vi "Sentuator_OS5000US.vi"(0 "VISA resource name":refnum<visa-resource-name>, 2 "Text to prepend to sentence":string="\n", 3 "error in (no error)":errorcluster) -> (4 "Angles":dbl[][](graph), 5 "VISA resource name out":refnum<visa-resource-name>, 6 "Remaining Sentence":string, 7 "error out":errorcluster)   [LabVIEW 2012]
uses:
  <instrlib>/Ocean Server OS4000/Ocean Server OS4000.lvlib
panel:
  in  "Send Output Rate":bool
  in  "Send Filter Value":bool
  in  "Send Mount Orientation":bool
  in  "Send Declination":bool
  in  "Output Rate":dbl
  in  "Average Samples":i32
  in  "Analog to Digital Conversion":i32
  in  "Mount Orientation (Default-Flat)":i32(ring)=1
  in  "Degauss Every":i32
  in  "Send Degauss":bool
  in  "Declination Angle":i32
  in  "Check Error":bool
  out "Error?":bool
  out "rollAngle":dbl
  out "pitchAngle":dbl
  out "compassHeading":dbl
  out "Mx":dbl
  out "My":dbl
  out "Mz":dbl
  out "Temperature":dbl
  out "Gyro X":dbl
  out "Gyro Y":dbl
  out "yAccel":dbl
  out "xAccel":dbl
  out "zAccel":dbl
  out "Magnetic Field":dbl[][](graph)
  out "Accel":dbl[][](graph)
  out "Temp":dbl[][](graph)
  out "Gyro":dbl[][](graph)
  out "Acceleration":dbl caption="Acceleration Magnitude"
  out "Magnetic Vector Field":dbl
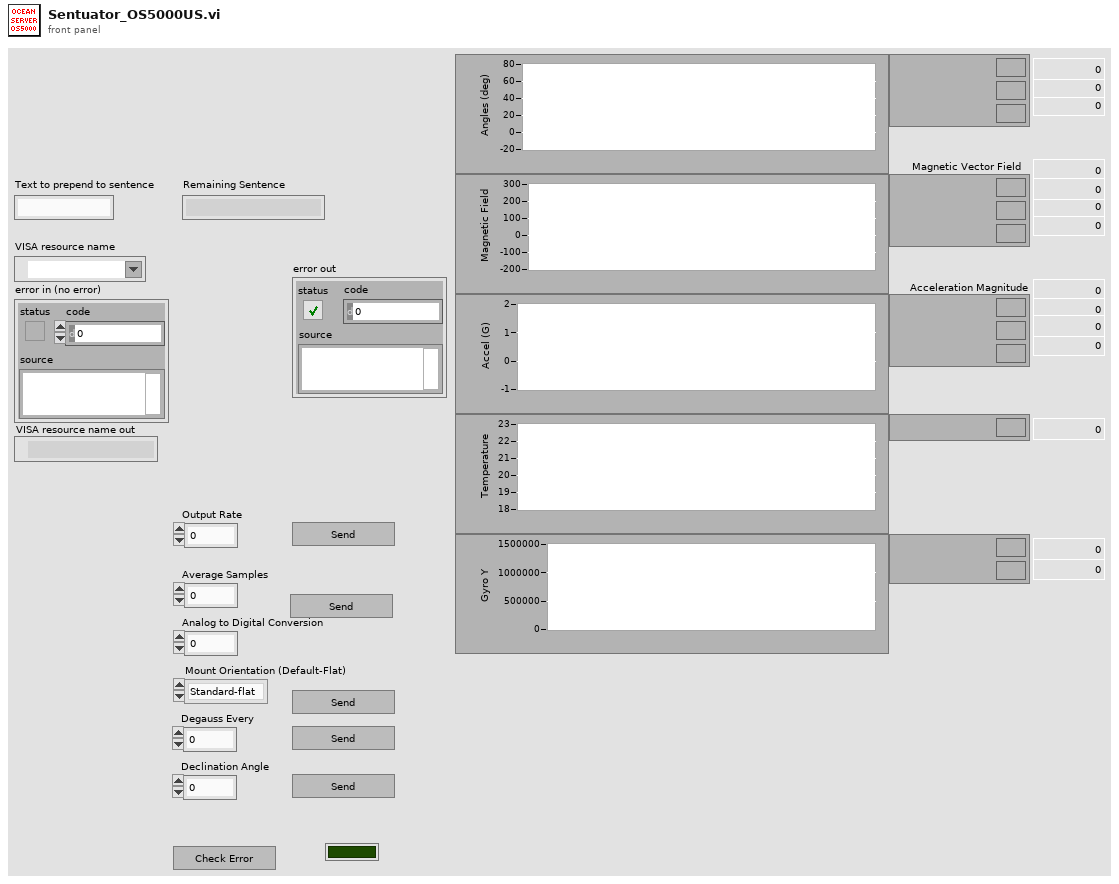
[diagram p1: front panel]
types:
  T1 = cluster{"Compass Heading":dbl, "pitch Angle":dbl, "roll Angle":dbl, "Temperature":dbl, "Depth":dbl, "Magnetic Field":dbl, "Magnetic Field X":dbl, "Magnetic Field Y":dbl, "Magnetic Field Z":dbl, "Acceleration":dbl, "Acceleration X":dbl, "Acceleration Y":dbl, "Gyro":dbl, "Gyro X":dbl, "Acceleration Z":dbl, "Gyro Y":dbl}
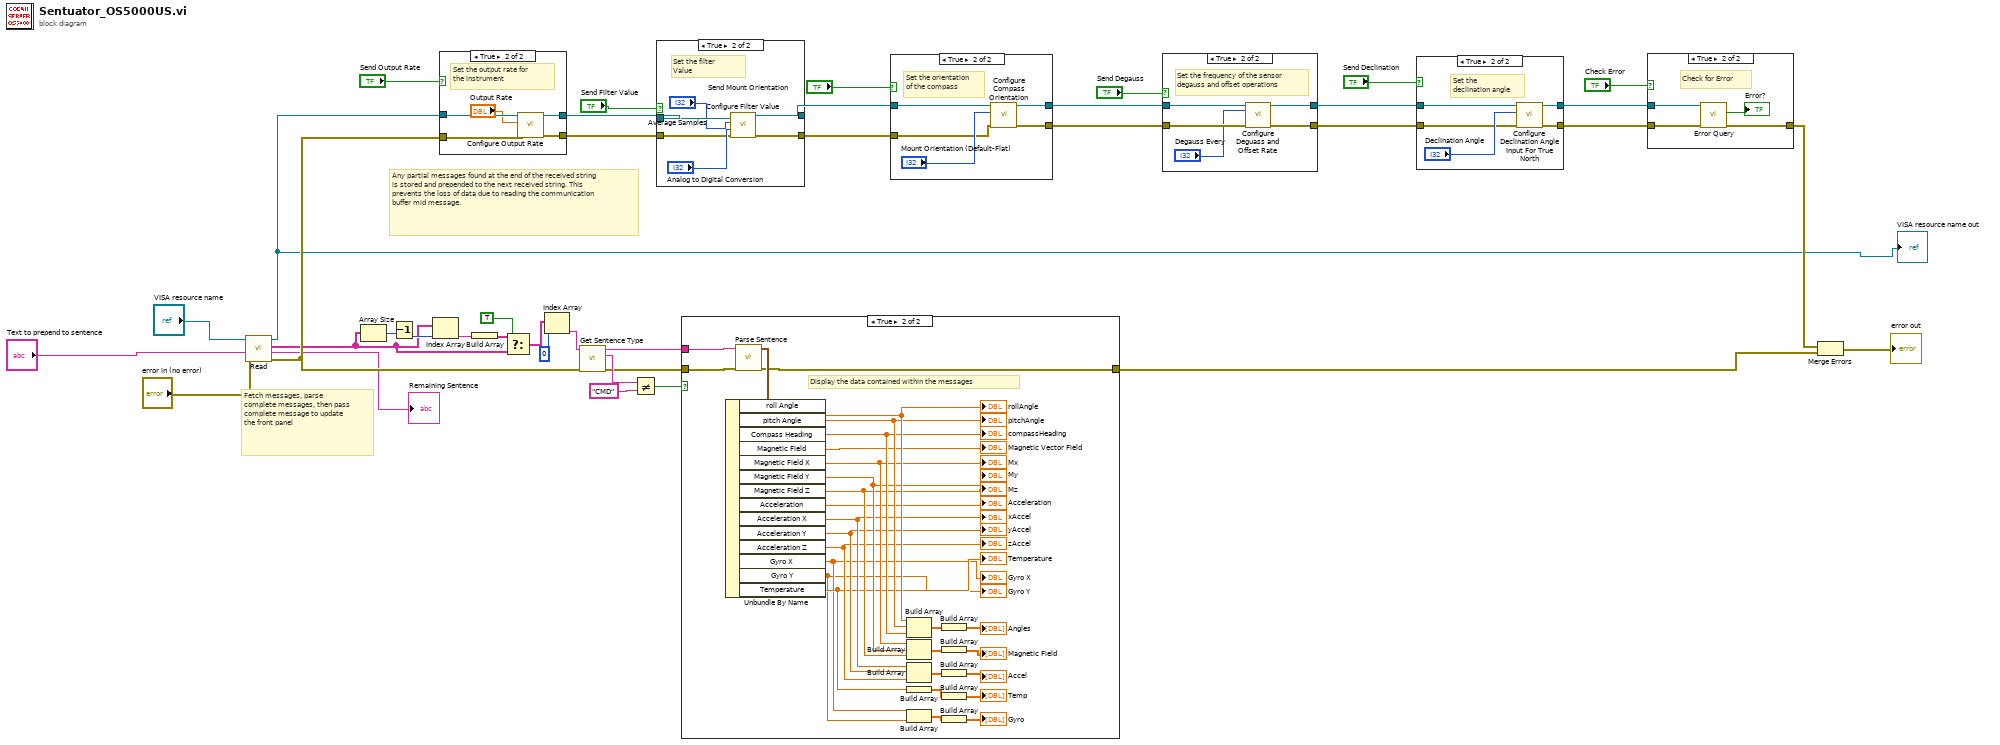
[diagram p0: block diagram]
diagram:
  # "Any partial messages found at the end of the received string is stored and prepended to the next received string. This prevents the loss of data due to reading the communication buffer mid message."
  # "Fetch messages, parse complete messages, then pass  complete message to update the front panel"
  n1 = call <instrlib>:"Read.vi"("error in (no error)"="error in (no error)", "Text to prepend to sentence"="Text to prepend to sentence", "VISA resource name"="VISA resource name") -> ("error out"=w27:errorcluster, "Remaining Sentence"=→"Remaining Sentence":string, "Ocean Server Sentences"=w16:string[], "VISA resource name out"=w7:refnum<visa-resource-name>)  [unwired: 5 in]
  "VISA resource name out" <- w7
  n2 = Array Size(array=w16) -> (size(s)=w20:i32)
  n3 = Decrement(x=w20) -> (x-1=w19:i32)
  n4 = Index Array(array=w16, index=w19) -> (element=w18:string)
  n5 = case shown="True" "Send Output Rate" {
    tunnel: w7 -> [w41 w46]
    tunnel: [w41 w44] -> w38
    tunnel: [w40 w43] -> w30
    tunnel: w27 -> [w40 w42]
    frame False {
    }
    frame True {
      # "Set the output rate for the instrument"
      n6 = call <instrlib>:"Configure Output Rate.vi"("Error in (no error)"=w42, "Output Rate ( 4 )"="Output Rate", "VISA resource name"=w46) -> ("Error out"=w43:errorcluster, "VISA resource out"=w44:refnum<visa-resource-name>)  [unwired: 7 in]
    }
  }
  n7 = Build Array(w18) -> (w17:string[])
  n8 = Select(t=w17, s=TRUE, f=w16) -> (s? t:f=w6:string[])
  n9 = Index Array(array=w6, index=0) -> (element=w4:string)
  n10 = call <instrlib>:"Get Sentence Type.vi"("error in (no error)"=w27, "Sentence In"=w4) -> ("error out"=w10:errorcluster, "Sentence Type"=w14:string, "Sentence Out"=w11:string)  [unwired: 7 in]
  n11 = Not Equal?(x=w14, y="CMD") -> (x != y?=w12:bool)
  n12 = case shown="True" "Send Filter Value" {
    tunnel: w38 -> [w48 w54]
    tunnel: [w48 w51] -> w36
    tunnel: w30 -> [w47 w50]
    tunnel: [w47 w49] -> w29
    frame False {
    }
    frame True {
      # "Set the filter Value"
      n13 = call <instrlib>:"Configure Filter Value.vi"("error in (no error)"=w50, "Filter Value for Analog to Digital Conversion ( 3 )"="Analog to Digital Conversion", "Averaging Value ( 4 )"="Average Samples", "VISA resource name"=w54) -> ("error out"=w49:errorcluster, "VISA resource out"=w51:refnum<visa-resource-name>)  [unwired: 6 in]
    }
  }
  n14 = case shown="True" w12 {
    tunnel: w11 -> [_ w59]
    tunnel: w10 -> [w55 w56]
    tunnel: [w55 w57] -> w21
    frame False {
      # "Front Panel isn't updated if the message received is not of the N1 type"
    }
    frame True {
      # "Display the data contained within the messages"
      n15 = call <instrlib>:"Parse Sentence.vi"("error in (no error)"=w56, "Ocean Server Sentence"=w59) -> ("error out"=w57:errorcluster, "Values"=w58:T1)  [unwired: 8 in]
      n16 = Unbundle By Name(w58) -> ("roll Angle"=w83:dbl, "pitch Angle"=w82:dbl, "Compass Heading"=w81:dbl, "Magnetic Field"=→"Magnetic Vector Field":dbl, "Magnetic Field X"=w80:dbl, "Magnetic Field Y"=w79:dbl, "Magnetic Field Z"=w78:dbl, "Acceleration"=→"Acceleration":dbl, "Acceleration X"=w77:dbl, "Acceleration Y"=w76:dbl, "Acceleration Z"=w75:dbl, "Gyro X"=w72:dbl, "Gyro Y"=w71:dbl, "Temperature"=w74:dbl)
      "rollAngle" <- w83
      "pitchAngle" <- w82
      "compassHeading" <- w81
      "Mx" <- w80
      "My" <- w79
      "Mz" <- w78
      "Temperature" <- w74
      "Gyro X" <- w72
      "Gyro Y" <- w71
      "yAccel" <- w76
      "xAccel" <- w77
      "zAccel" <- w75
      n17 = Build Array(w83, w82, w81) -> (w67:dbl[])
      n18 = Build Array(w80, w79, w78) -> (w68:dbl[])
      n19 = Build Array(w77, w76, w75) -> (w69:dbl[])
      n20 = Build Array(w74) -> (w73:dbl[])
      n21 = Build Array(w72, w71) -> (w70:dbl[])
      n22 = Build Array(w67) -> (→"Angles":dbl[][])
      n23 = Build Array(w68) -> (→"Magnetic Field":dbl[][])
      n24 = Build Array(w69) -> (→"Accel":dbl[][])
      n25 = Build Array(w73) -> (→"Temp":dbl[][])
      n26 = Build Array(w70) -> (→"Gyro":dbl[][])
    }
  }
  n27 = case shown="True" "Send Mount Orientation" {
    tunnel: w36 -> [w85 w89]
    tunnel: [w85 w88] -> w34
    tunnel: w29 -> [w84 w87]
    tunnel: [w84 w86] -> w28
    frame False {
    }
    frame True {
      # "Set the orientation of the compass"
      n28 = call <instrlib>:"Configure Compass Orientation.vi"("error in (no error)"=w87, "Mount Orientation ( Flat )"="Mount Orientation (Default-Flat)", "VISA resource name"=w89) -> ("error out"=w86:errorcluster, "VISA resource out"=w88:refnum<visa-resource-name>)  [unwired: 7 in]
    }
  }
  n29 = case shown="True" "Send Degauss" {
    tunnel: w34 -> [w92 w97]
    tunnel: [w92 w96] -> w33
    tunnel: [w91 w95] -> w32
    tunnel: w28 -> [w91 w94]
    frame False {
    }
    frame True {
      # "Set the frequency of the sensor degauss and offset operations"
      n30 = call <instrlib>:"Configure Deguass and Offset Rate.vi"("error in (no error)"=w94, "Deguass and Offset Rate ( 1 )"="Degauss Every", "VISA resource name"=w97) -> ("error out"=w95:errorcluster, "VISA resource out"=w96:refnum<visa-resource-name>)  [unwired: 7 in]
    }
  }
  n31 = case shown="True" "Send Declination" {
    tunnel: w33 -> [w99 w103]
    tunnel: w32 -> [w98 w102]
    tunnel: [w99 w101] -> w25
    tunnel: [w98 w100] -> w24
    frame False {
    }
    frame True {
      # "Set the declination angle"
      n32 = call <instrlib>:"Configure Declination Angle Input For True North.vi"("error in (no error)"=w102, "Declination Angle ( 0 degrees)"="Declination Angle", "VISA resource name"=w103) -> ("error out"=w100:errorcluster, "VISA resource out"=w101:refnum<visa-resource-name>)  [unwired: 7 in]
    }
  }
  n33 = case shown="True" "Check Error" {
    tunnel: w25 -> [_ w109]
    tunnel: w24 -> [w105 w108]
    tunnel: [w105 w106] -> w23
    frame False {
    }
    frame True {
      # "Check for Error"
      n34 = call <instrlib>:"Error Query.vi"("error in (no error)"=w108, "VISA resource name"=w109) -> ("error out"=w106:errorcluster, "Error"=→"Error?":bool)  [unwired: 7 in, 1 out]
    }
  }
  n35 = Merge Errors(w23, w21) -> (→"error out":errorcluster)
